vi "Global.vi"() -> ()   [LabVIEW 2014]
panel:
  in  "count":i32
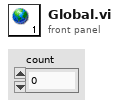
[diagram p1: front panel]
diagram:
